vi "GetConnected.vi"(11 "MB_MODULE in":refnum<class "MB_MODULE.lvclass">) -> (2 "Connected":bool)   [LabVIEW 2019, in "MB_MODULE.lvclass"]
uses:
  MB_MODULE.lvclass
  MB_MODULE.lvclass/MB_MODULE.ctl
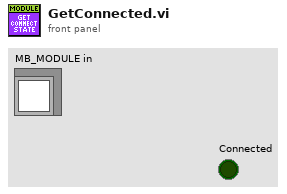
[diagram p1: front panel]
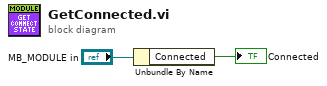
[diagram p0: block diagram]
diagram:
  n1 = Unbundle By Name("MB_MODULE in") -> ("Connected"=→"Connected":bool)
